vi "write_access_codes_to_file.vi"(8 "error in (no error)":errorcluster, 9 "Cluster":T1, 11 "Path":path) -> (0 "error out":errorcluster)   [LabVIEW 2016]
uses:
  <vilib>/Utility/config.llb/Write Key (String).vi
  <vilib>/Utility/config.llb/NI_LVConfig.lvlib
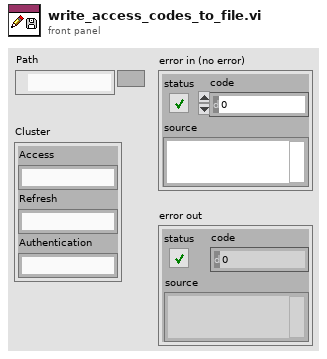
[diagram p1: front panel]
types:
  T1 = cluster{"Access":string, "Refresh":string, "Authentication":string}
  T2 = typedef "NI_LVConfig.lvlib/Config Data RefNum.ctl" = refnum<k1>
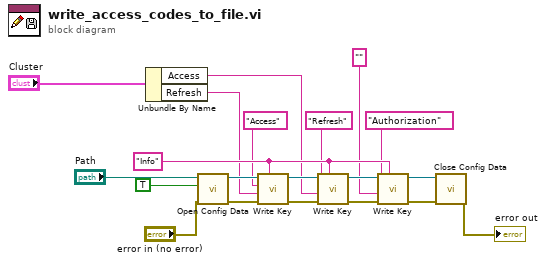
[diagram p0: block diagram]
diagram:
  w13 = "Info"
  n1 = Unbundle By Name("Cluster") -> ("Access"=w3:string, "Refresh"=w2:string)
  n2 = call <vilib>:"Open Config Data.vi"("error in (no error)"="error in (no error)", "create file if necessary (T)"=TRUE, "configuration file path"="Path") -> ("error out"=w19:errorcluster, "refnum"=w17:T2)  [unwired: 6 in, 1 out]
  n3 = call-poly <vilib>:"Write Key.vi"("section"=w13, "error in (no error)"=w19, "value"=w2, "key"="Access", "refnum"=w17) -> ("error out"=w18:errorcluster, "refnum out"=w16:T2)  [unwired: 4 in, 1 out]
  n4 = call-poly <vilib>:"Write Key.vi"("section"=w13, "error in (no error)"=w18, "value"=w3, "key"="Refresh", "refnum"=w16) -> ("error out"=w15:errorcluster, "refnum out"=w14:T2)  [unwired: 4 in, 1 out]
  n5 = call-poly <vilib>:"Write Key.vi"("section"=w13, "error in (no error)"=w15, "value"="", "key"="Authorization", "refnum"=w14) -> ("error out"=w11:errorcluster, "refnum out"=w12:T2)  [unwired: 4 in, 1 out]
  n6 = call <vilib>:"Close Config Data.vi"("error in (no error)"=w11, "refnum"=w12) -> ("error out"=→"error out":errorcluster)  [unwired: 8 in, 1 out]
